vi "Update INI key to users last set value.vi"(6 "Don't allow empty directorys (true)":bool, 8 "error in (no error)":errorcluster, 9 "Directory Path":path, 10 "INI Key":string, 11 "INI Section":string) -> (0 "error out":errorcluster, 1 "Created Directory Path":path)   [LabVIEW 2010]
doc: "Makes Sure path is up to date, changes directory per users input, updates INI to reflect change"
uses:
  <vilib>/Utility/sysdir.llb/System Directory Type.ctl
  <vilib>/Utility/config.llb/Write Key (Path).vi
  <vilib>/Utility/config.llb/NI_LVConfig.lvlib
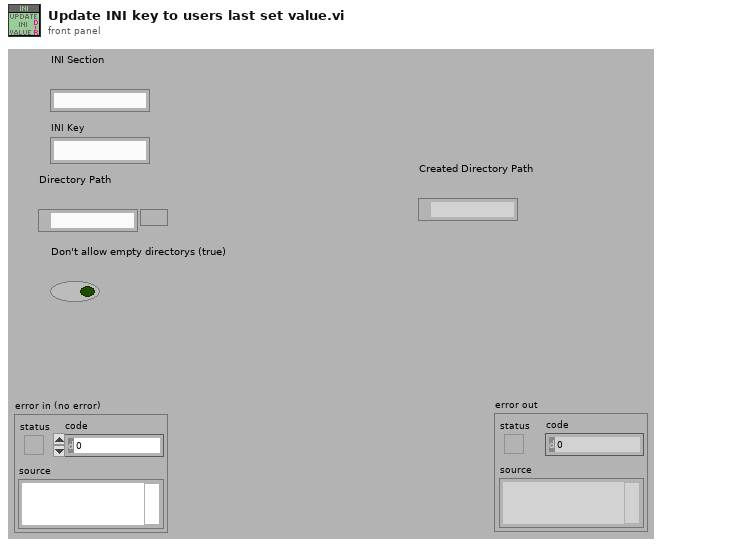
[diagram p1: front panel]
types:
  T1 = typedef "System Directory Type.ctl" = i32
  T2 = typedef "NI_LVConfig.lvlib/Config Data RefNum.ctl" = refnum<k1>
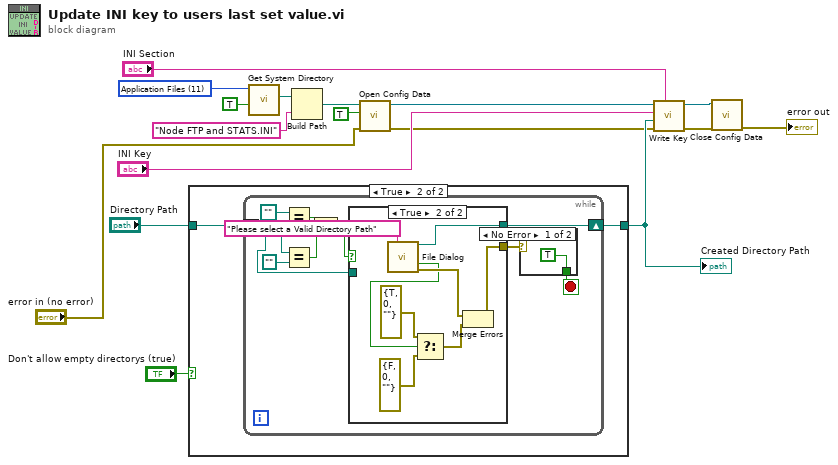
[diagram p0: block diagram]
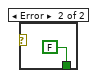
[diagram p3: hidden frame]
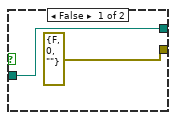
[diagram p4: hidden frame]
diagram:
  w8 = T1 11 items=["User Home"=0, "User Desktop"=1, "User Documents"=2, "User Application Data"=3, "User Preferences"=4, "User Temporary"=5, "Public Documents"=6, "Public Application Data"=7, "Public Preferences"=8, "Public Cache"=13, "System Core Libraries"=9, "System Installed Libraries"=10, "Application Files"=11, "Boot Volume Root"=12] ("system directory type")
  n1 = case shown="True" "Don't allow empty directorys (true)" {
    tunnel: [w18 w20] -> w13
    tunnel: "Directory Path" -> [w18 w19]
    frame False {
    }
    frame True {
      n2 = while {
        shift-right: [w23] -> w20
        shift-left: w19 -> [w24]
        stop <- w21 stop-if-true
        n3 = Equal?(x=path "", y=w24) -> (x = y?=w27:bool)
        n4 = Equal?(x=w24, y=path "") -> (x = y?=w26:bool)
        n5 = Compound Arithmetic op=OR(w27, w26) -> (w25:bool)
        n6 = case shown="True" w25 {
          tunnel: w24 -> [w33 _]
          tunnel: [w33 w41] -> w23
          tunnel: [errorcluster {"status"=FALSE, "code"=0, "source"=""} ("error out") w34] -> w22
          frame False {
          }
          frame True {
            n7 = call "File Dialog"("prompt"="Please select a Valid Directory Path") -> ("selected path"=w41:path, "cancelled"=w35:bool, "error out"=w36:errorcluster)  [unwired: 11 in, 1 out]
            n8 = Select(t=errorcluster {"status"=TRUE, "code"=0, "source"=""} ("error in"), s=w35, f=errorcluster {"status"=FALSE, "code"=0, "source"=""} ("error in")) -> (s? t:f=w37:errorcluster)
            n9 = Merge Errors(w36, w37) -> (w34:errorcluster)
          }
        }
        n10 = case shown="No Error" w22 {
          tunnel: [TRUE FALSE] -> w21
          frame No Error {
          }
          frame Error {
          }
        }
      }
    }
  }
  "Created Directory Path" <- w13
  n11 = call <vilib>:"Get System Directory.vi"("create directory if not found? (F)"=TRUE, "system directory type"=w8) -> ("system directory"=w9:path)  [unwired: 9 in]
  n12 = Build Path(base path=w9, name or relative path="Node FTP and STATS.INI") -> (appended path=w11:path)
  n13 = call <vilib>:"Open Config Data.vi"("error in (no error)"="error in (no error)", "create file if necessary (T)"=TRUE, "configuration file path"=w11) -> ("error out"=w3:errorcluster, "refnum"=w5:T2)  [unwired: 6 in, 1 out]
  n14 = call-poly <vilib>:"Write Key.vi"("section"="INI Section", "error in (no error)"=w3, "value"=w13, "key"="INI Key", "refnum"=w5) -> ("error out"=w2:errorcluster, "refnum out"=w12:T2)  [unwired: 4 in, 1 out]
  n15 = call <vilib>:"Close Config Data.vi"("error in (no error)"=w2, "refnum"=w12) -> ("error out"=→"error out":errorcluster)  [unwired: 8 in, 1 out]
